vi "VI-Layout XControl Facade.vi"(0 "VI":path, 11 "error in (no error)":errorcluster) -> (15 "error out":errorcluster)   [LabVIEW 2015]
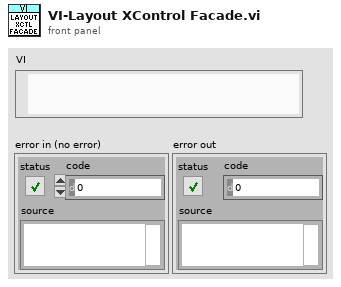
[diagram p1: front panel]
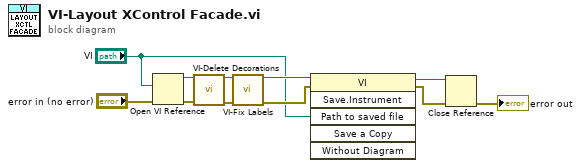
[diagram p0: block diagram]
diagram:
  n1 = Open VI Reference(vi path="VI", error in (no error)="error in (no error)") -> (vi reference=w8:refnum<vi>, error out=w11:errorcluster)  [unwired: 4 in]
  n2 = call "VI-Delete Decorations.vi"("VI in"=w8, "error in (no error)"=w11) -> ("VI out"=w10:refnum<vi>, "error out"=w9:errorcluster)  [unwired: 12 in]
  n3 = call "VI-Fix Labels.vi"("VI in"=w10, "error in (no error)"=w9) -> ("VI out"=w5:refnum<vi>, "error out"=w4:errorcluster)  [unwired: 12 in]
  n4 = invoke class="VI" method="Save.Instrument"(reference=w5, error in=w4, "Path to saved file"="VI") -> (reference out=w2:refnum<vi>, error out=w3:errorcluster)  [unwired: 3 in, 4 out]
  n5 = Close Reference(reference=w2, error in (no error)=w3) -> (error out=→"error out":errorcluster)
